vi "Query inputs.vi"(8 "error in (no error)":errorcluster, 11 "VISA resource name":refnum<visa-resource-name>) -> (0 "error out":errorcluster, 1 "T=?":T1, 2 "B=?":T1, 3 "VISA resource name out":refnum<visa-resource-name>, 4 "Externally-triggered?":bool, 5 "A=?":T1)   [LabVIEW 2017, in "SR400.lvlib"]
doc: "CI i { ,j }\nThe CI command sets and reads the counter\ninputs. i = 0, 1, or 2 selecting counter A,B, or T\nand is required. If j is included, then the input to\ncounter i is changed to source j. If j is absent, the\ninput to counter i is returned.\n\nj Input\n0 10 MHz\n1 INPUT 1\n2 INPUT 2\n3 TRIG\n\nCounter Allowed Inputs\nA-- 10 MHz, INPUT1\nB --INPUT 1, INPUT 2\nT --10 MHz, INPUT 2, TRIG\n\nChanging a counter input while counting may\nresult in bad count data"
uses:
  SR400.lvlib
  Typedefs.llb/Counting Input.ctl
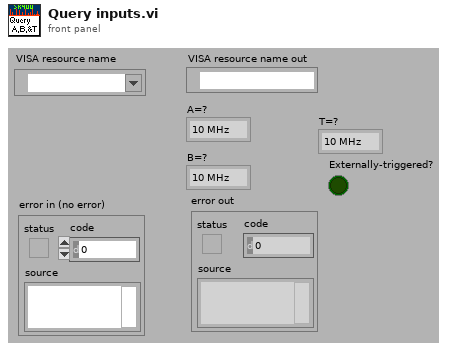
[diagram p1: front panel]
types:
  T1 = typedef "SR400.lvlib/Counting Input.ctl" = enum16{"10 MHz", "INPUT 1", "INPUT 2", "TRIG"}
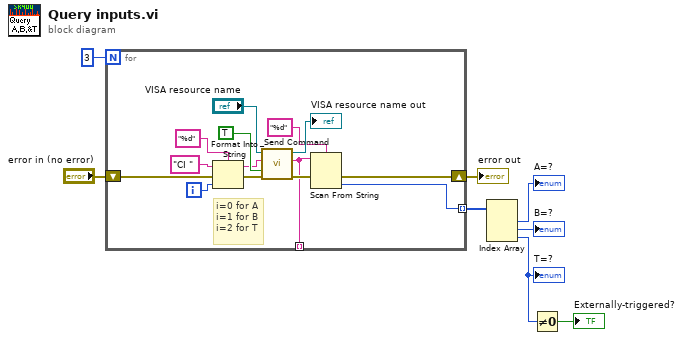
[diagram p0: block diagram]
diagram:
  n1 = for {
    N: 3 -> [_]
    tunnel: [w12] -> w8 mode=indexing
    shift-right: [w13] -> w5
    shift-left: "error in (no error)" -> [w11]
    tunnel: [w9] -> _ mode=indexing
    i -> [w10]
    # "i=0 for A\ni=1 for B\ni=2 for T"
    n2 = Format Into String(format string="%d", initial string="CI " ("command"), error in=w11, w10) -> (resulting string=w18:string, error out=w19:errorcluster)
    n3 = call "_Send Command.vi"("error in (no error)"=w19, "Query? (F)"=TRUE, "Command"=w18, "VISA resource name"="VISA resource name") -> ("error out"=w21:errorcluster, "Response"=w9:string, "VISA resource name out"=→"VISA resource name out":refnum<visa-resource-name>)  [unwired: 5 out]
    n4 = Scan From String(format string="%d", input string=w9, error in=w21) -> (error out=w13:errorcluster, output 1=w12:i32)  [unwired: 1 in, 3 out]
  }
  "error out" <- w5
  n5 = Index Array(array=w8) -> (element #1=→"A=?":i32, element #2=→"B=?":i32, element #3=w3:i32)  [unwired: 3 in]
  "T=?" <- w3
  n6 = Not Equal To 0?(x=w3) -> (x != 0?=→"Externally-triggered?":bool)
